vi "Launch Tasks.vi"(8 "error in (no error)":errorcluster, 11 "Series Actor in":refnum<class "Series Actor.lvclass">) -> (0 "error out":errorcluster, 3 "Series Actor out":refnum<class "Series Actor.lvclass">)   [LabVIEW 2023, in "Series Actor.lvlib" / "Series Actor.lvclass"]
uses:
  Series Actor.lvclass
  Series Actor.lvclass/Series Actor.ctl
  Series Base/Series Base.lvclass
  <vilib>/ActorFramework/Actor/Actor.lvclass
  Task Actor/Task Actor/Task Actor/Task Actor.lvclass
  C:/Program Files/National Instruments/LabVIEW 2023/vi.lib/ActorFramework/Actor/Actor.lvclass
  D:/git/HAL/HAL GOOP4/Task Actor/Task Actor/Task Actor/Task Actor.lvclass
  D:/git/HAL/HAL GOOP4/Series Actor/Series Actor/Series Actor.lvclass
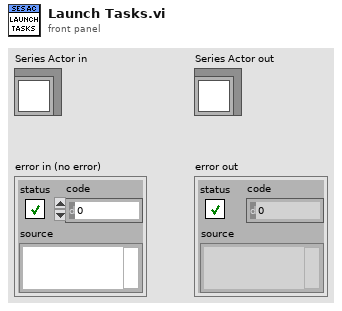
[diagram p1: front panel]
types:
  T1 = map{string, refnum<class "Message Enqueuer.lvclass">}
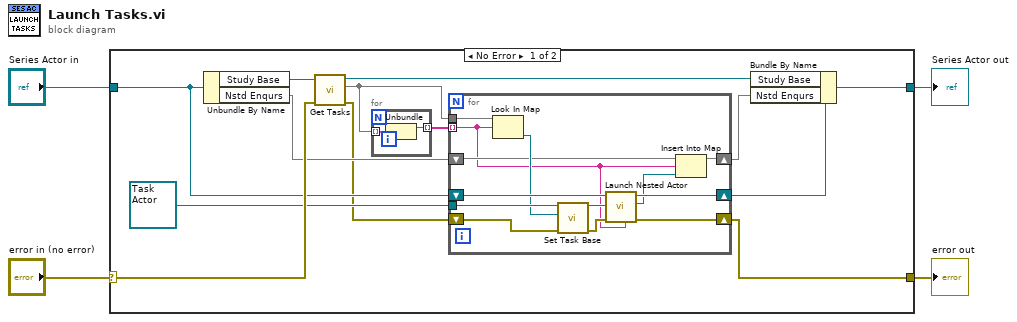
[diagram p0: block diagram]
diagram:
  n1 = case shown="No Error" "error in (no error)" {
    selector: "error in (no error)" -> [w16 w34]
    tunnel: [w15 w34] -> w3
    tunnel: [w17 w33] -> w1
    tunnel: "Series Actor in" -> [w13 w33]
    frame No Error {
      n2 = Unbundle By Name(w13) -> ("Study Base"=w12:refnum<class "Series Base.lvclass">, "Nstd Enqurs"=w8:T1)
      n3 = call "Get Tasks.vi"("error in (no error)"=w16, "HAL GOOP4:Series Base in"=w12) -> ("error out"=w7:errorcluster, "Tasks"=w9:map{string, refnum<class "Task Base.lvclass">}, "HAL GOOP4:Series Base out"=w11:refnum<class "Series Base.lvclass">)  [unwired: 7 in]
      n4 = for {
        tunnel: w9 -> [w32] mode=indexing
        tunnel: [w31] -> w10 mode=indexing
        n5 = Unbundle(w32) -> (w31:string)  [unwired: 1 out]
      }
      n6 = for {
        tunnel: w10 -> [w18] mode=indexing
        tunnel: w9 -> [w30]
        tunnel: refnum<class "Task Actor.lvclass"> refnum ("Task Actor.lvlib:Task Actor.lvclass") -> [w28]
        shift-right: [w25] -> w5
        shift-left: w13 -> [w29]
        shift-right: [w22] -> w6
        shift-left: w8 -> [w24]
        shift-right: [w19] -> w15
        shift-left: w7 -> [w21]
        n7 = Look In Map(map=w30, key=w18) -> (value=w26:refnum<class "Task Base.lvclass">)  [unwired: 1 in, 1 out]
        n8 = call "Set Task Base.vi"("error in (no error)"=w21, "HAL GOOP4.lvlib:Task Base.lvclass"=w26, "Task Actor in"=w28) -> ("error out"=w20:errorcluster, "Task Actor out"=w27:refnum<class "Task Actor.lvclass">)  [unwired: 7 in]
        n9 = call <vilib>:"Launch Nested Actor.vi"("Debug Alias"=w18, "error in (no error)"=w20, "Nested Actor"=w27, "Caller Actor in"=w29) -> ("error out"=w19:errorcluster, "Nested Actor's Enqueuer"=w23:refnum<class "Message Enqueuer.lvclass">, "Caller Actor out"=w25:refnum<class "Series Actor.lvclass">)  [unwired: 5 in]
        n10 = Insert Into Map(map in=w24, key=w18, value=w23) -> (map out=w22:T1)  [unwired: 2 out]
      }
      n11 = Bundle By Name(cluster=w5, "Study Base"=w11, "Nstd Enqurs"=w6) -> (w17:refnum<class "Series Actor.lvclass">)
    }
    frame Error {
    }
  }
  "error out" <- w3
  "Series Actor out" <- w1
